vi "Colormap to Array.vi"(10 "Min Pressure":dbl, 11 "Max Pressure":dbl) -> (3 "Z Scale.Marker Values[]":cluster{dbl, u32}[](array[cluster]))   [LabVIEW 2021]
panel:
  out "Color Array":u32[](array[numeric])
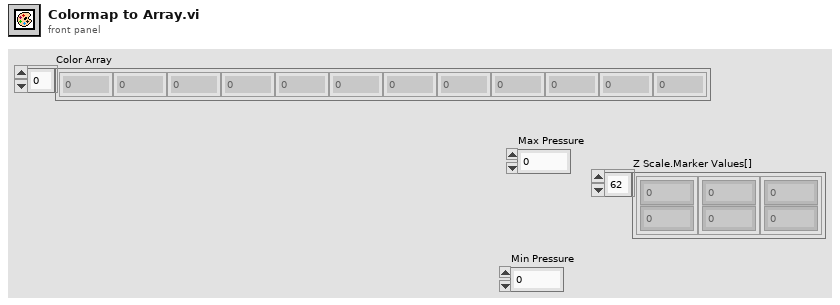
[diagram p1: front panel]
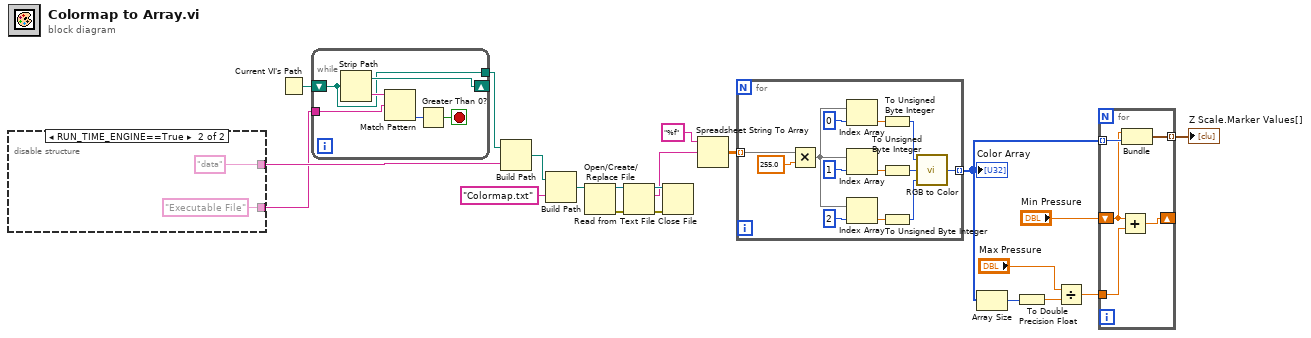
[diagram p0: block diagram]
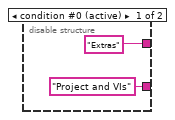
[diagram p2: hidden frame]
diagram:
  n1 = disable-structure shown="RUN_TIME_ENGINE==True" {
    disable-tunnel: ["Extras" ("name or relative path") "data" ("name or relative path")] -> w5
    disable-tunnel: ["Project and VIs" ("regular expression") "Executable File" ("regular expression")] -> w1
    frame condition #0 (active) {
    }
    frame condition #1 {
    }
  }
  n2 = Current VI's Path() -> (path=w3:path)
  n3 = while {
    shift-right: [w28] -> _
    shift-left: w3 -> [w27]
    tunnel: [w27] -> w2
    tunnel: w1 -> [w26]
    stop <- w29 stop-if-true
    n4 = Strip Path(path=w27) -> (stripped path=w28:path, name=w31:string)
    n5 = Match Pattern(string=w31, regular expression=w26) -> (offset past match=w30:i32)  [unwired: 1 in, 3 out]
    n6 = Greater Than 0?(x=w30) -> (x > 0?=w29:bool)
  }
  n7 = Build Path(base path=w2, name or relative path=w5) -> (appended path=w4:path)
  n8 = Build Path(base path=w4, name or relative path="Colormap.txt") -> (appended path=w7:path)
  n9 = Open/Create/Replace File(file path (use dialog)=w7) -> (refnum out=w20:refnum<file>, error out=w21:errorcluster)  [unwired: 5 in, 1 out]
  n10 = Read from Text File(file (use dialog)=w20, error in=w21) -> (refnum out=w19:refnum<file>, text=w16:string, error out=w18:errorcluster)  [unwired: 2 in, 1 out]
  n11 = Close File(refnum=w19, error in=w18) -> ()  [unwired: 2 out]
  n12 = Spreadsheet String To Array(format string="%f", spreadsheet string=w16) -> (array=w15:dbl[][])  [unwired: 2 in]
  n13 = for {
    tunnel: w15 -> [w44] mode=indexing
    tunnel: [w32] -> w14 mode=indexing
    n14 = Multiply(x=w44, y=255.0) -> (x*y=w42:dbl[])
    n15 = Index Array(array=w42, index=0) -> (element=w37:dbl)
    n16 = Index Array(array=w42, index=1) -> (element=w35:dbl)
    n17 = Index Array(array=w42, index=2) -> (element=w36:dbl)
    n18 = To Unsigned Byte Integer(number=w37) -> (unsigned 8bit integer=w38:u8)
    n19 = To Unsigned Byte Integer(number=w35) -> (unsigned 8bit integer=w34:u8)
    n20 = To Unsigned Byte Integer(number=w36) -> (unsigned 8bit integer=w33:u8)
    n21 = call <vilib>:"RGB to Color.vi"("B"=w33, "G"=w34, "R"=w38) -> ("Color"=w32:u32)
  }
  "Color Array" <- w14
  n22 = Array Size(array=w14) -> (size(s)=w12:i32)
  n23 = To Double Precision Float(number=w12) -> (double precision float=w11:dbl)
  n24 = Divide(x="Max Pressure", y=w11) -> (x/y=w9:dbl)
  n25 = for {
    tunnel: w14 -> [w49] mode=indexing
    shift-right: [w48] -> _
    shift-left: "Min Pressure" -> [w47]
    tunnel: w9 -> [w46]
    tunnel: [w45] -> w8 mode=indexing
    n26 = Add(x=w47, y=w46) -> (x+y=w48:dbl)
    n27 = Bundle("Min Pressure"=w47, "Color"=w49) -> (w45:cluster{"Min Pressure":dbl, "Color":u32})  [unwired: 1 in]
  }
  "Z Scale.Marker Values[]" <- w8
